vi "Zad1.vi"() -> ()   [LabVIEW 2018]
panel:
  out "Results For":i32[](array[numeric])
  out "Results While":i32[](array[numeric])
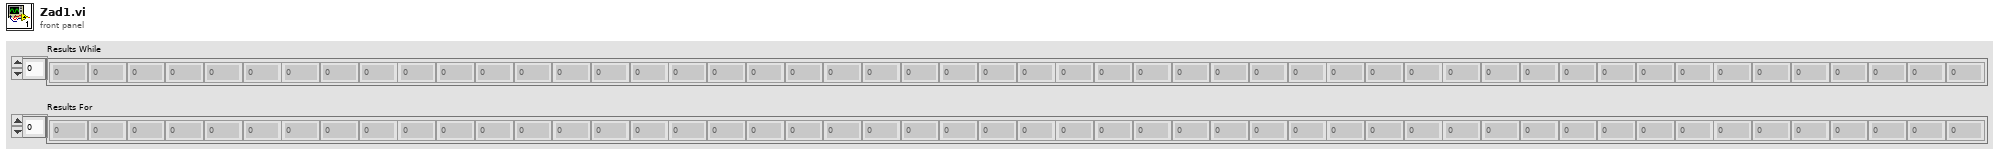
[diagram p1: front panel]
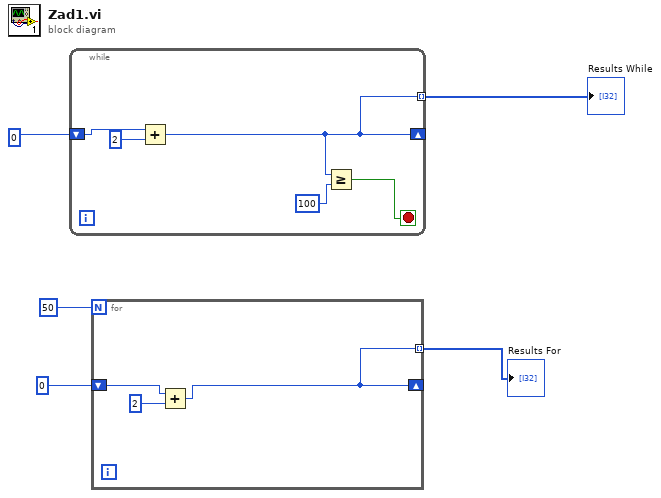
[diagram p0: block diagram]
diagram:
  n1 = while {
    shift-right: [w7] -> _
    shift-left: 0 -> [w6]
    tunnel: [w7] -> w5 mode=indexing
    stop <- w9 stop-if-true
    n2 = Add(x=w6, y=2) -> (x+y=w7:i32)
    n3 = Greater Or Equal?(x=w7, y=100) -> (x >= y?=w9:bool)
  }
  "Results While" <- w5
  n4 = for {
    N: 50 -> [_]
    shift-right: [w11] -> _
    shift-left: 0 -> [w12]
    tunnel: [w11] -> w1 mode=indexing
    n5 = Add(x=w12, y=2) -> (x+y=w11:i32)
  }
  "Results For" <- w1
